vi "Replace Array Subset (Multi).vi"(5 "JSON Array":refnum<class "JSON Value.lvclass">, 9 "index":i32, 11 "new element/subarray":refnum<class "JSON Value.lvclass">[](array[class])) -> (6 "output JSON Array":refnum<class "JSON Value.lvclass">)   [LabVIEW 2016, in "JSON Value.lvclass"]
doc: "Replaces an element or subarray in an array at the point you specify in index."
uses:
  JSON Value.lvclass
  JSON Value.lvclass/JSON Value.ctl
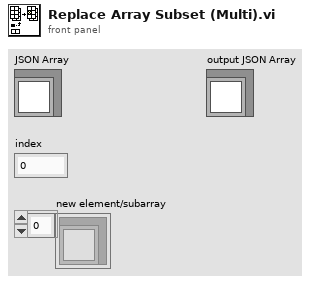
[diagram p1: front panel]
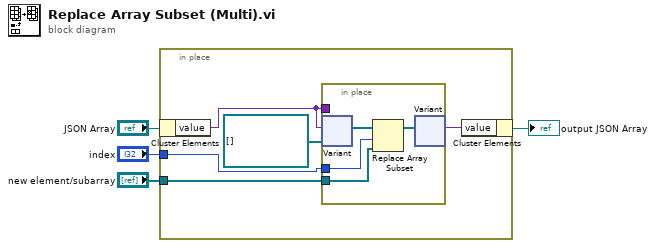
[diagram p0: block diagram]
diagram:
  n1 = in-place {
    in-place-border: "new element/subarray" -> [w9]
    in-place-border: "index" -> [w8]
    n2 = in-place-cluster #1("JSON Array") -> ("value"=w7:variant)
    n3 = in-place {
      in-place-border: w9 -> [w13]
      in-place-border: w8 -> [w12]
      in-place-border: w7 -> [_]
      n4 = in-place-variant #2(w7, refnum<class "JSON Value.lvclass">[] [] ("output array")) -> (w11:refnum<class "JSON Value.lvclass">[])  [unwired: 1 out]
      n5 = Replace Array Subset(array=w11, new element=w13, index=w12) -> (w10:refnum<class "JSON Value.lvclass">[])
      n6 = in-place-variant #2(w10) -> (w5:variant)  [unwired: 1 out]
    }
    n7 = in-place-cluster #1("value"=w5) -> (→"output JSON Array":refnum<class "JSON Value.lvclass">)
  }
